vi "test-out.vi"() -> ()   [LabVIEW 2017]
panel:
  out "Value":dbl
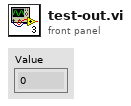
[diagram p1: front panel]
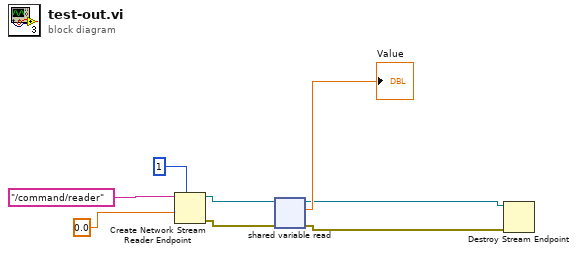
[diagram p0: block diagram]
diagram:
  n1 = Create Network Stream Reader Endpoint(7:1 ("reader buffer size"), 9:0.0, 11:"/command/reader" ("reader name")) -> (0:w4:errorcluster, 3:w5:refnum<k21>)  [unwired: 4 in]
  n2 = shared-variable-read(w5, w4) -> (w2:refnum<k21>, w1:errorcluster, →"Value":dbl)  [unwired: 1 in, 1 out]
  n3 = Destroy Stream Endpoint(8:w1, 11:w2) -> ()  [unwired: 1 out]
